vi "Write Paths.vi"(8 "error in (no error)":errorcluster, 10 "Paths":T1, 11 "WebView2 Control in":refnum<class "WebView2 Control.lvclass">) -> (0 "error out":errorcluster, 3 "WebView2 Control out":refnum<class "WebView2 Control.lvclass">)   [LabVIEW 2020, in "WebView2.lvlib" / "WebView2 Control.lvclass"]
uses:
  WebView2 Control.lvclass
  Paths.ctl
  WebView2 Control.lvclass/WebView2 Control.ctl
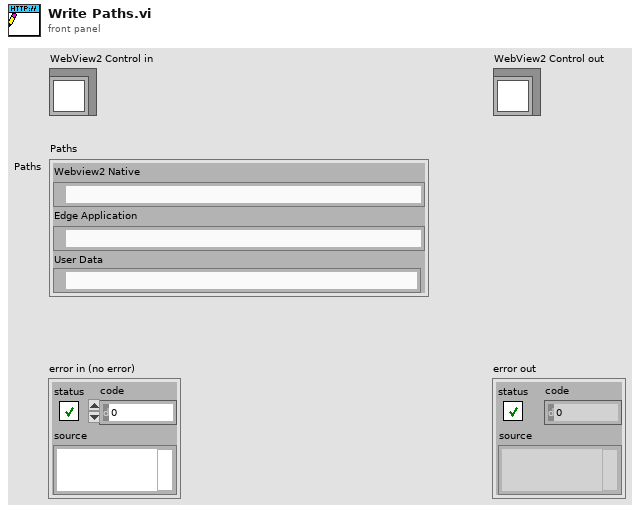
[diagram p1: front panel]
types:
  T1 = typedef "WebView2.lvlib/WebView2 Control.lvclass/Paths.ctl" = cluster{"Webview2 Native":path, "Edge Application":path, "User Data":path}
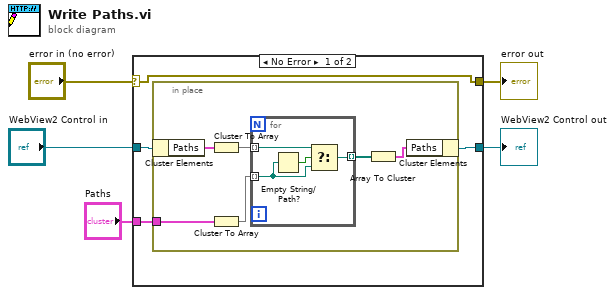
[diagram p0: block diagram]
diagram:
  n1 = case shown="No Error" "error in (no error)" {
    selector: "error in (no error)" -> [w9 w20]
    tunnel: [w9 w20] -> w4
    tunnel: [w7 w21] -> w2
    tunnel: "WebView2 Control in" -> [w8 w21]
    tunnel: "Paths" -> [w6 _]
    frame No Error {
      n2 = in-place {
        in-place-border: w6 -> [w10]
        n3 = in-place-cluster #1(w8) -> ("Paths"=w12:T1)
        n4 = Cluster To Array(cluster=w12) -> (array=w13:path[])
        n5 = Cluster To Array(cluster=w10) -> (array=w15:path[])
        n6 = for {
          tunnel: [w19] -> w14 mode=indexing
          tunnel: w13 -> [w16] mode=indexing
          tunnel: w15 -> [w17] mode=indexing
          n7 = Empty String/Path?(string/path=w17) -> (empty?=w18:bool)
          n8 = Select(t=w16, s=w18, f=w17) -> (s? t:f=w19:path)
        }
        n9 = Array To Cluster(array=w14) -> (cluster=w11:cluster{"[0]":path, "[1]":path, "[2]":path})
        n10 = in-place-cluster #1("Paths"=w11) -> (w7:refnum<class "WebView2 Control.lvclass">)
      }
    }
    frame Error {
    }
  }
  "error out" <- w4
  "WebView2 Control out" <- w2
